vi "Main.vi"(8 "error in (no error)":errorcluster, 11 "Test_ExampleClassA in":refnum<class "Test_ExampleClassA.lvclass">) -> (0 "error out":errorcluster, 3 "Test_ExampleClassA out":refnum<class "Test_ExampleClassA.lvclass">)   [LabVIEW 2012, in "Test_ExampleClassA.lvclass"]
doc: "Main VI and GUI of the component class. Performs the unit test of ExampleClassA."
uses:
  Test_ExampleClassA.lvclass
  ExampleClassA/ExampleClassA.lvclass
  MurmexTest/Set test subject.vi
  Murmex/Set configure at initialise.vi
  MurmexTest/Set number of tests.vi
  MurmexTest/Set default tests.vi
  Murmex/Murmex.lvclass
panel:
  in  "component ID":string
  # "Instructions\n\nThis is the unit test component for ExampleClassA.\n\n- Configure an instance of the test subject (ExampleClassA) to have this unit test component as an observer.\n\n- Configure an instance of this unit test component to have above-mentioned instance of ExampleClassA as the test subject.\n\nStart the unit test component instance and the test subject instance either manually (in that case, enter their respective IDs on their GUIs) or via the ServiceManager."
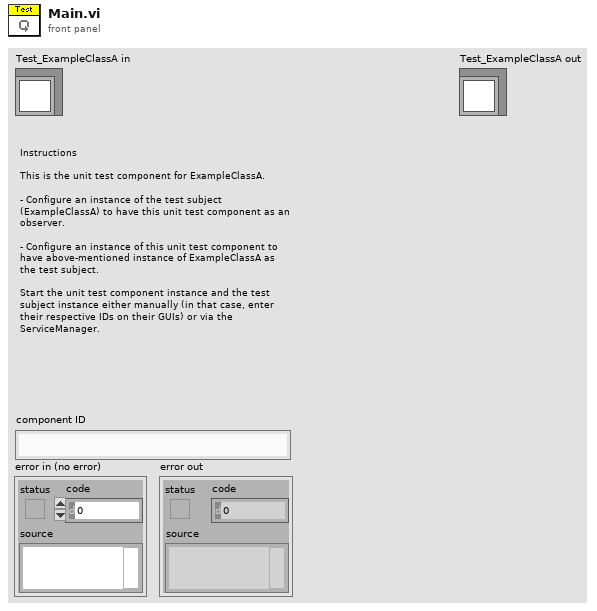
[diagram p1: front panel]
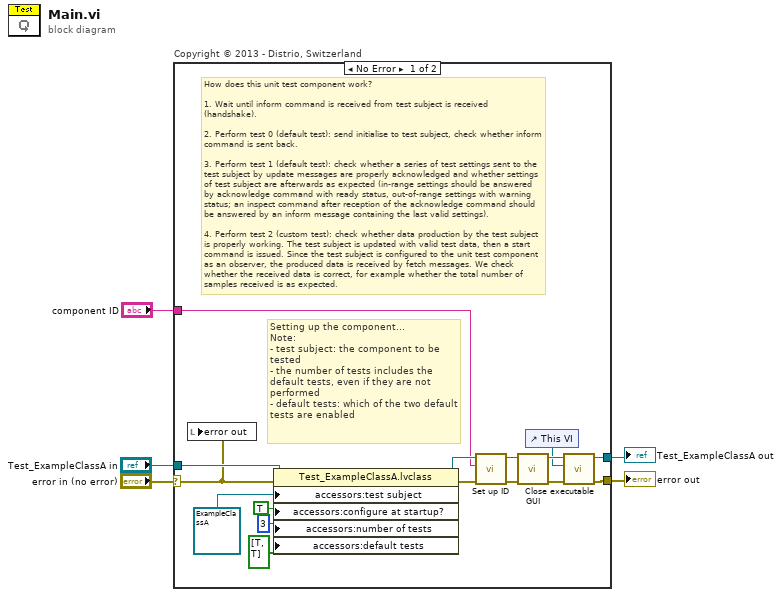
[diagram p0: block diagram]
diagram:
  n1 = case "Copyright © 2013 - Distrio, Switzerland" shown="No Error" "error in (no error)" {
    selector: "error in (no error)" -> [w17 w23]
    tunnel: "Test_ExampleClassA in" -> [w21 w22]
    tunnel: [w9 w23] -> w3
    tunnel: [w7 w22] -> w2
    tunnel: "component ID" -> [w12 _]
    frame No Error {
      # "How does this unit test component work?\n\n1. Wait until inform command is received from test subject is received (handshake).\n\n2. Perform test 0 (default test): send initialise to test subject, check whether inform command is sent back.\n\n3. Perform test 1 (default test): check whether a series of test settings sent to the test subject by update messages are properly acknowledged and whether settings of test subject are afterwards as expected (in-range settings should be answered by acknowledge command with ready status, out-of-range settings with warning status; an inspect command after reception of the acknowledge command should be answered by an inform message containing the last valid settings).\n\n4. Perform test 2 (custom test): check whether data production by the test subject is properly working. The test subject is updated with valid test data, then a start command is issued. Since the test subject is configured to the unit test component as an observer, the produced data is received by fetch messages. We check whether the received data is correct, for example whether the total number of samples received is as expected."
      # "Setting up the component...\nNote:\n- test subject: the component to be tested\n- the number of tests includes the default tests, even if they are not performed\n- default tests: which of the two default tests are enabled"
      n2 = local write "error out"(w17) -> ()
      n3 = property class="Test_ExampleClassA.lvclass"(reference=w21, error in=w17, "accessors:test subject"=refnum<class "ExampleClassA.lvclass"> refnum ("ExampleClassA.lvclass"), "accessors:configure at startup?"=TRUE ("configure at startup?"), "accessors:number of tests"=3 ("number of tests"), "accessors:default tests"=bool[] [TRUE, TRUE] ("default tests")) -> (reference out=w18:refnum<class "Test_ExampleClassA.lvclass">, error out=w19:errorcluster)
      n4 = call "Set up ID.vi"("error in (no error)"=w19, "component ID"=w12, "MurmexBase in"=w18) -> ("error out"=w14:errorcluster, "MurmexBase out"=w13:refnum<class "Test_ExampleClassA.lvclass">)  [unwired: 6 in, 1 out]
      n5 = call-dynamic "GUI.vi"("error in (no error)"=w14, "MurmexTest in"=w13) -> ("error out"=w10:errorcluster, "MurmexTest out"=w8:refnum<class "Test_ExampleClassA.lvclass">)  [unwired: 8 in]
      n6 = control-ref of="This VI"() -> (w6:refnum<vi>)
      n7 = call "Close executable.vi"("error in (no error)"=w10, "main VI ref (optional)"=w6, "MurmexBase in"=w8) -> ("error out"=w9:errorcluster, "MurmexBase out"=w7:refnum<class "Test_ExampleClassA.lvclass">)  [unwired: 7 in]
    }
    frame Error {
    }
  }
  "error out" <- w3
  "Test_ExampleClassA out" <- w2
